vi "Setting-DC.vi"(6 "error in (no error)":errorcluster caption="错误输入（无错误）", 7 "簇":T1, 8 "极化时间":dbl, 9 "极化电压":dbl, 10 "极化温度":dbl, 11 "变温速率":dbl) -> (0 "剩余时间":dbl, 1 "当前电压":bool, 2 "当前温度":dbl, 3 "极化完毕":bool, 4 "error out":errorcluster caption="错误输出")   [LabVIEW 2017]
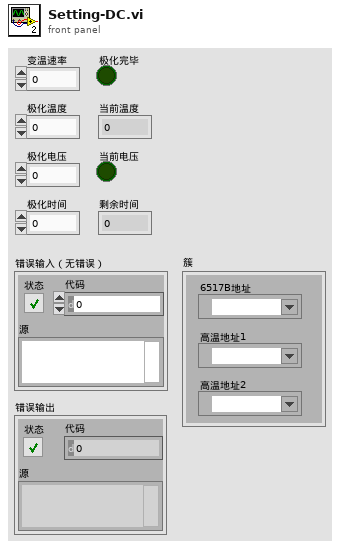
[diagram p1: front panel]
types:
  T1 = cluster{"6517B地址":refnum<visa-resource-name>, "高温地址1":refnum<visa-resource-name>, "高温地址2":refnum<visa-resource-name>}
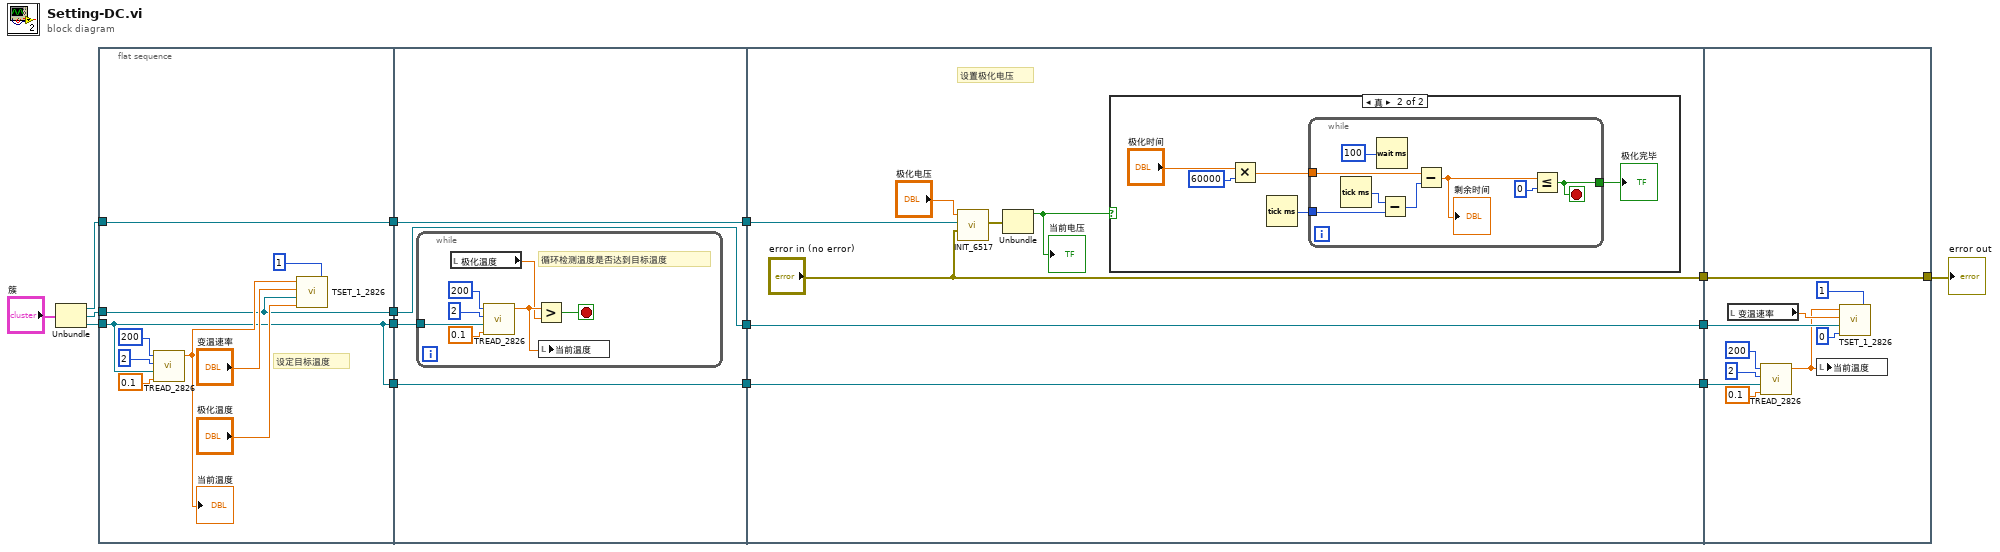
[diagram p0: block diagram]
diagram:
  n1 = Unbundle("簇") -> ("6517B地址"=w9:refnum<visa-resource-name>, "高温地址1"=w13:refnum<visa-resource-name>, "高温地址2"=w14:refnum<visa-resource-name>)
  n2 = flat-sequence {
    tunnel: w14 -> [w16]
    tunnel: w13 -> [w17]
    tunnel: [w16] -> w12
    tunnel: [w18] -> w10
    tunnel: w9 -> [w18]
    tunnel: [w17] -> w4
    tunnel: [w16] -> w1
    tunnel: w12 -> [w29]
    tunnel: [w28] -> w11
    tunnel: w10 -> [w28]
    tunnel: [w27] -> w5
    tunnel: w4 -> [w27]
    tunnel: [w26] -> w2
    tunnel: w1 -> [w26]
    tunnel: w11 -> [w42]
    tunnel: ["error in (no error)"] -> w7
    tunnel: [w38] -> w6
    tunnel: w5 -> [w38]
    tunnel: [w37] -> w3
    tunnel: w2 -> [w37]
    tunnel: [w66] -> w8
    tunnel: w7 -> [w66]
    tunnel: w6 -> [w65]
    tunnel: w3 -> [w59]
    frame #0 {
      # "设定目标温度"
      n3 = call "TREAD_2826.vi"("Unknown Param 2"=0.1, "VISA resource name"=w16, "Address No."=2, "Unknown Param"=200) -> ("PV"=w21:dbl)  [unwired: 3 out]
      "当前温度" <- w21
      n4 = call "TSET_1_2826.vi"("Address No."=i8 1, "T-Ending, C"="极化温度", "VISA resource name"=w17, "cooling/heating rate, C/min"="变温速率", "T-Starting, C"=w21) -> ()
    }
    frame #1 {
      n5 = while {
        tunnel: w29 -> [w34]
        stop <- w30 stop-if-true
        # "循环检测温度是否达到目标温度"
        n6 = local read "极化温度"() -> (w31:dbl)
        n7 = call "TREAD_2826.vi"("Unknown Param 2"=0.1, "VISA resource name"=w34, "Address No."=2, "Unknown Param"=200) -> ("PV"=w32:dbl)  [unwired: 3 out]
        n8 = Greater?(x=w32, y=w31) -> (0:w30:bool)
        n9 = local write "当前温度"(w32) -> ()
      }
    }
    frame #2 {
      # "设置极化电压"
      n10 = call "INIT_6517.vi"("error in (no error)"="error in (no error)", "VISA resource name"=w42, "Vin"="极化电压") -> ("error out"=w41:errorcluster)  [unwired: 7 in, 1 out]
      n11 = Unbundle(w41) -> ("status"=w40:bool)  [unwired: 2 out]
      "当前电压" <- w40
      n12 = case shown="真" w40 {
        frame False {
        }
        frame True {
          n13 = Multiply(x="极化时间", y=60000) -> (x*y=w45:dbl)
          n14 = Tick Count (ms)() -> (millisecond timer value=w46:u32)
          n15 = while {
            tunnel: w46 -> [w55]
            tunnel: w45 -> [w54]
            tunnel: [w49] -> w44
            stop <- w49 stop-if-true
            n16 = Tick Count (ms)() -> (millisecond timer value=w56:u32)
            n17 = Wait (ms)(milliseconds to wait=100) -> ()  [unwired: 1 out]
            n18 = Subtract(x=w56, y=w55) -> (x-y=w53:u32)
            n19 = Subtract(x=w54, y=w53) -> (x-y=w52:dbl)
            "剩余时间" <- w52
            n20 = Less Or Equal?(x=w52, y=0) -> (x <= y?=w49:bool)
          }
          "极化完毕" <- w44
        }
      }
    }
    frame #3 {
      n21 = local read "变温速率"() -> (w62:dbl)
      n22 = call "TREAD_2826.vi"("Unknown Param 2"=0.1, "VISA resource name"=w59, "Address No."=2, "Unknown Param"=200) -> ("PV"=w57:dbl)  [unwired: 3 out]
      n23 = local write "当前温度"(w57) -> ()
      n24 = call "TSET_1_2826.vi"("Address No."=i8 1, "T-Ending, C"=0, "VISA resource name"=w65, "cooling/heating rate, C/min"=w62, "T-Starting, C"=w57) -> ()
    }
  }
  "error out" <- w8
